vi "Experiment header-Get typedef cluster ref.vi"(7 "Header file sections":T22, 8 "error in (no error)":errorcluster, 11 "All header parameters / Header module interface cluster":refnum<vi>) -> (0 "error out":errorcluster, 1 "All header parameters in 2":refnum<vi>, 2 "Section Refs":T21[](array[typedef]), 3 "Controls[]":refnum<vi>[](array[refnum]))   [LabVIEW 2020]
uses:
  Typedefs/Header file sections.ctl
  Typedefs/Header file section refs.ctl
  Typedefs/Header parameters cluster-ALL.ctl
  Typedefs/Header subclusters/Header params -Login.ctl
  Typedefs/Header subclusters/Header params-Global Parameters.ctl
  Misc/Experiment Type.ctl
  Typedefs/Header subclusters/Header params-Imaging Modes.ctl
  Typedefs/Header subclusters/Header params-Time Series.ctl
  Typedefs/Header subclusters/Header params-Basic image meta data.ctl
  Typedefs/Frame Size.ctl
  Typedefs/Header subclusters/Header params-Motor Z-stack.ctl
  Typedefs/Header subclusters/Header params-AOL Z-stack.ctl
  Typedefs/Header subclusters/Header params-Functional Imaging.ctl
  Typedefs/Functional Mode.ctl
  Typedefs/AOL modes.ctl
  Typedefs/Plane Mode.ctl
  Typedefs/Header subclusters/Header params-Movement correction.ctl
  Typedefs/Reference source.ctl
  Typedefs/Header subclusters/Header params-Calibration Setup.ctl
  Typedefs/Header subclusters/Header params-statistics.ctl
  Misc/Biology Information.ctl
  Typedefs/Header subclusters/Header params-calibration data.ctl
panel:
  in  "All header parameters in":T1 {"VOLUME IMAGING"."Plane Mode" items=["XY Plane", "XZ Plane", "YZ Plane", "arbitraryplane"]; "VOLUME IMAGING"."Basic Image meta data"."Frame Size" items=["100X100"=100, "128X128"=128, "200X200"=200, "256X256"=256, "512X512"=512, "1024x1024"=1024, "2048x2048"=2048]; "AOL Z-STACK"."Hdr Basic Image meta data"."Frame Size" items=["100X100"=100, "128X128"=128, "200X200"=200, "256X256"=256, "512X512"=512, "1024x1024"=1024, "2048x2048"=2048]; "MOTOR Z-STACK"."Hdr Basic Image meta data"."Frame Size" items=["100X100"=100, "128X128"=128, "200X200"=200, "256X256"=256, "512X512"=512, "1024x1024"=1024, "2048x2048"=2048]; "FUNCTIONAL IMAGING"."Plane Mode" items=["XY Plane", "XZ Plane", "YZ Plane", "arbitraryplane"]; "FUNCTIONAL IMAGING"."Basic Image meta data"."Frame Size" items=["100X100"=100, "128X128"=128, "200X200"=200, "256X256"=256, "512X512"=512, "1024x1024"=1024, "2048x2048"=2048]; "TIME SERIES"."Basic Image meta data"."Frame Size" items=["100X100"=100, "128X128"=128, "200X200"=200, "256X256"=256, "512X512"=512, "1024x1024"=1024, "2048x2048"=2048]}
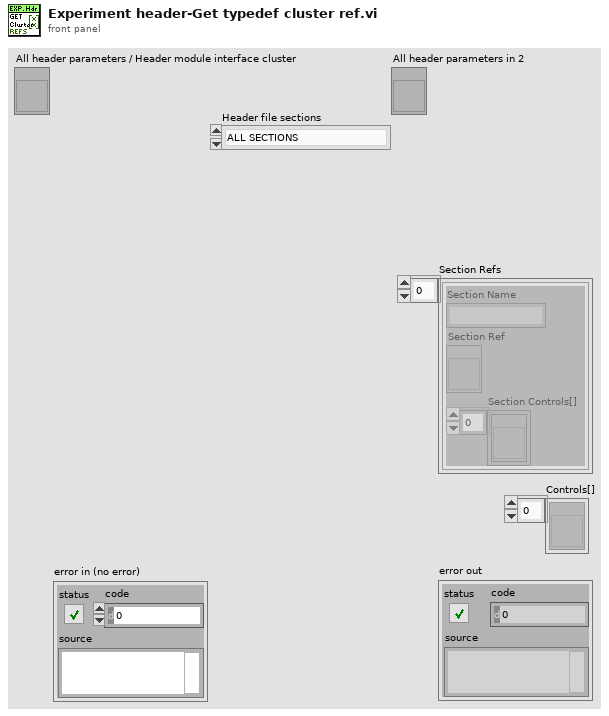
[diagram p1: front panel]
types:
  T1 = typedef "Header parameters cluster-ALL.ctl" = cluster{"LOGIN":T2, "GLOBAL PARAMETERS":T3, "IMAGING MODES":T5, "TIME SERIES":T6, "MOTOR Z-STACK ":T9, "AOL Z-STACK":T10, "FUNCTIONAL IMAGING":T11, "VOLUME IMAGING":T11, "MOVEMENT CORRECTION":T15, "CALIBRATION":T17, "STATISTICS":T18, "BIOLOGY INFORMATION":T19, "Calibration Data":T20}
  T2 = typedef "Header params -Login.ctl" = cluster{"User":string, "Profile":string, "Software Version":string, "Experiment Date Time":timestamp}
  T3 = typedef "Header params-Global Parameters.ctl" = cluster{"MicroscopeID":string, "Microscope Type":string, "Objective":string, "Field of View (um)":dbl, "Fill time (us)":dbl, "Experiment Type":T4, "Stimuli Trigger":bool, "Speed Logging":bool}
  T4 = typedef "Experiment Type.ctl" = enum16{"In vivo", "In vitro", "Testing", "Calibration", "Other"}
  T5 = typedef "Header params-Imaging Modes.ctl" = cluster{"Time Series":bool, "Motor Zstack":bool, "AOL Zstack":bool, "Functional Imaging":bool, "Volume Imaging":bool}
  T6 = typedef "Header params-Time Series.ctl" = cluster{"Basic Image meta data":T7, "AOL z":dbl}
  T7 = typedef "Header params-Basic image meta data.ctl" = cluster{"Wavelength (nm)":dbl, "# averaged frames":dbl, "laser power (%)":dbl, "Pockels":dbl, "pixel dwell time (us)":dbl, "pmt 1":dbl, "pmt 2":dbl, "back apperture":dbl, "zoom":dbl, "field of view":dbl, "Frame Size":T8, "AOL x centre":dbl, "AOL y centre":dbl, "Stage x position":dbl, "Stage y position":dbl, "Stage z position":dbl}
  T8 = typedef "Frame Size.ctl" = u16
  T9 = typedef "Header params-Motor Z-stack.ctl" = cluster{"Hdr Basic Image meta data":T7, "Z Start":dbl, "Z Stop":dbl, "No of Planes":i32, "Laser Power (%) at Z Start":dbl, "Laser Power (%) at Z Stop":dbl}
  T10 = typedef "Header params-AOL Z-stack.ctl" = cluster{"Hdr Basic Image meta data":T7, "Z Start":dbl, "Z Stop":dbl, "No of Planes":i32, "Laser Power (%) at Z Start":dbl, "Laser Power (%) at Z Stop":dbl}
  T11 = typedef "Header params-Functional Imaging.ctl" = cluster{"Functional Mode":T12, "Variable Length":bool, "Variable Resolution":bool, "Pockels Modulation":bool, "Stimuli Trigger":bool, "Cool down enabled":bool, "AOL Mode":T13, "Plane Mode":T14, "Miniscan Dwell time per pixel (us)":dbl, "poi dwell time":dbl, "Number of trials":dbl, "Number of cycles":dbl, "Number of pois":dbl, "Number of miniscans":dbl, "Number of pixels in miniscan":dbl, "Rectangle ROI length":dbl, "Rectangle ROI height":dbl, "Frame rate (fps)":dbl, "Acquisition Length":dbl, "video length (sec)":dbl, "Stimuli delay (sec)":dbl, "Cool down time (sec)":dbl, "Basic Image meta data":T7, "Z Start (um)":dbl, "Z Stop (um)":dbl}
  T12 = typedef "Functional Mode.ctl" = enum16{"Point", "Line", "Patch", "Plane", "Volume"}
  T13 = typedef "AOL modes.ctl" = enum16{"Raster", "Structural", "Pointing", "Mini Scan", "Alignment"}
  T14 = typedef "Plane Mode.ctl" = u16
  T15 = typedef "Header params-Movement correction.ctl" = cluster{"Movement Correction":bool, "Axial Reference":bool, "Reference Source":T16, "Full Frame Size":dbl, "Reference Field of View":dbl, "Reference Zoom":dbl, "Reference dwell time (us)":dbl, "Reference X Pixels":dbl, "Reference Y Pixels":dbl, "Number of Z lines":dbl, "Size of Z pixels":dbl, "Axial Pixels":dbl, "Ignore Z lines":dbl, "Reference Scan Cycles":dbl, "Reference Threshold XY":dbl, "Reference Threshold Z":dbl, "Reference Average XY":dbl, "Reference Average Z":dbl, "Proportional Scale":dbl, "Integral Scale":dbl, "Proportional Scale Z":dbl, "Integral Scale Z":dbl, "Diff Threshold":dbl, "Diff Threshold Z":dbl, "Sliding Average":bool, "Reference count reset enabled":bool, "Scan Interval (ms)":dbl, "Ref Plot Refresh Rate (ms)":dbl}
  T16 = typedef "Reference source.ctl" = enum16{"Green channel", "Red channel"}
  T17 = typedef "Header params-Calibration Setup.ctl" = cluster{"Pockels Calibration File":path, "Calibration_ini file":path, "Setup_ini file":path}
  T18 = typedef "Header params-statistics.ctl" = cluster{"Z-stack duration (sec)":dbl, "Number of acquired data-points":dbl, "Acquisition time (ms)":dbl, "Number of acquired frames":dbl, "Intertrial times":dbl[]}
  T19 = typedef "Biology Information.ctl" = cluster{"Animal Code or Name":string, "Animal DoB":string, "Animal Age":string, "Animal Sex":string, "Animal Weight":string, "Date of Injection":string, "Date of Implant":string, "Site of Injection":string, "Animal Ear Notch":string, "AAV constructs":string, "Genetic background":string, "Optical reporter":string, "Region of brain imaged":string, "Other \ncomments":string}
  T20 = typedef "Header params-calibration data.ctl" = cluster{"Objective Name":string, "Calibration Wavelength":dbl, "Sum X":dbl, "Sum Y":dbl, "Diff X":dbl, "Diff Y":dbl, "Distortion Correction":dbl, " Z norm to um Scaling":dbl, " X norm to um Scaling":dbl}
  T21 = typedef "Header file section refs.ctl" = cluster{"Section Name":string, "Section Ref":refnum<vi>, "Section Controls[]":refnum<vi>[]}
  T22 = typedef "Header file sections.ctl" = enum16{"ALL SECTIONS", "LOGIN", "GLOBAL PARAMETERS", "CALIBRATION DATA", "IMAGING MODES", "TIME SERIES", "MOTOR Z-STACK", "AOL Z-STACK", "FUNCTIONAL IMAGING", "VOLUME IMAGING", "ARBOREAL SCANNING", "MULTIBEAM PARAMETERS", "MOVEMENT CORRECTION", "CALIBRATION", "STATISTICS", "BIOLOGY INFORMATION", "PARAMETER SWEEP"}
  T23 = cluster{"Label.Text":string, refnum<vi>, "Controls OUT":refnum<vi>[]}
  T24 = cluster{"Label.Text":string, refnum<vi>, "Controls OUT":refnum<vi>[]}[]
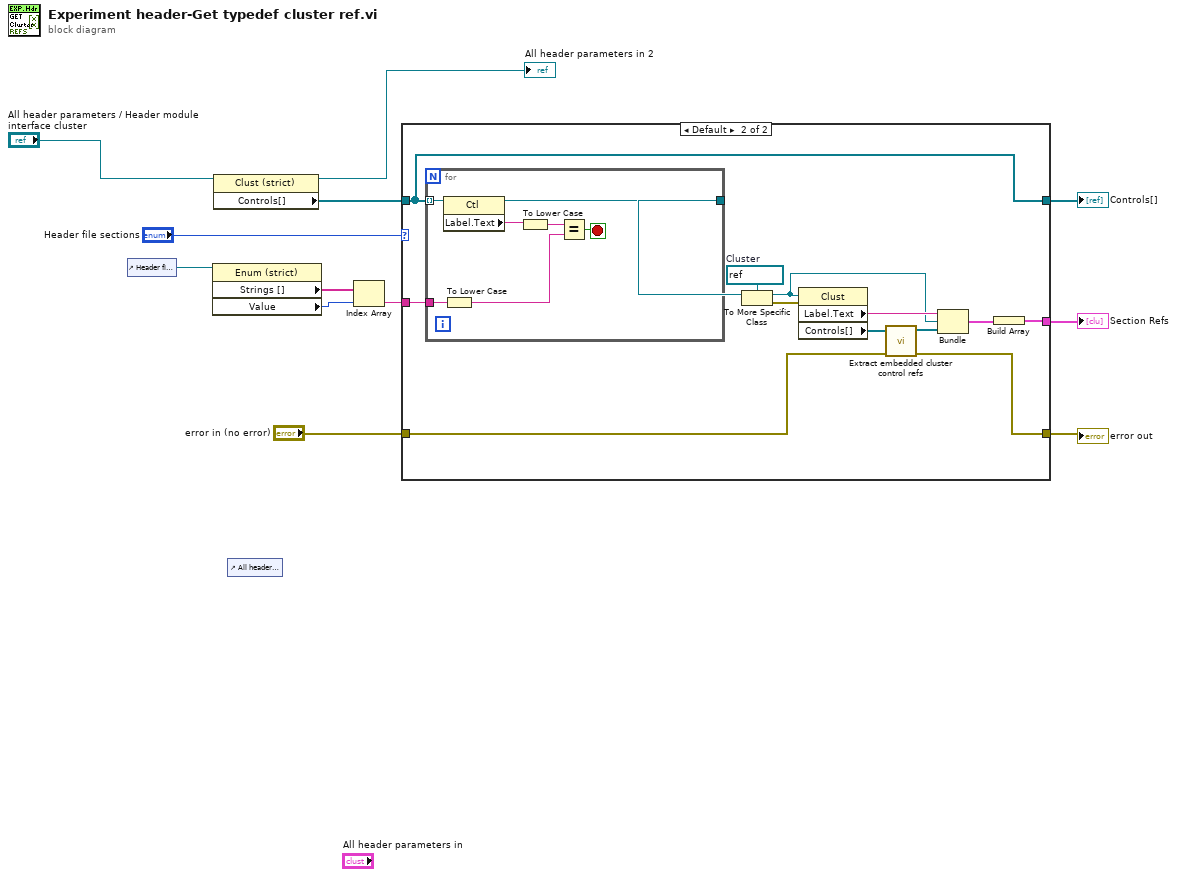
[diagram p0: block diagram]
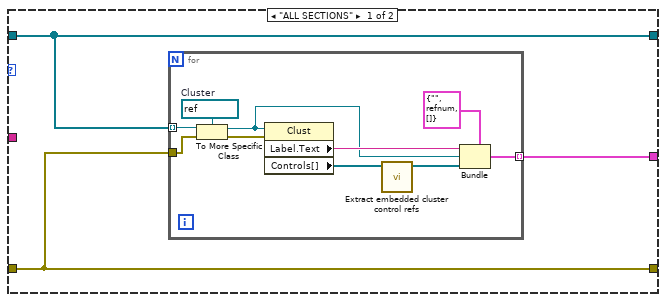
[diagram p2: hidden frame]
diagram:
  n1 = control-ref of="Header file sections"() -> (w9:refnum<vi>)
  n2 = property on="Property Node" class="Enum (strict)"(reference=w9) -> ("Strings []"=w8:string[], "Value"=w7:T22)  [unwired: 1 in, 2 out]
  n3 = property on="Property Node" class="Clust (strict)"(reference="All header parameters / Header module interface cluster") -> (reference out=→"All header parameters in 2":refnum<vi>, "Controls[]"=w11:refnum<vi>[])  [unwired: 1 in, 1 out]
  n4 = control-ref of="All header parameters in"() -> ()  [unwired: 1 out]
  n5 = Index Array(array=w8, index=w7) -> (element=w6:string)
  n6 = case shown="Default" "Header file sections" {
    tunnel: w11 -> [w15 w37]
    tunnel: [w15 w37] -> w10
    tunnel: w6 -> [_ w38]
    tunnel: "error in (no error)" -> [w14 w27]
    tunnel: [w14 w26] -> w4
    tunnel: [w13 w30] -> w3
    frame "ALL SECTIONS" {
      n7 = for {
        tunnel: w15 -> [w25] mode=indexing
        tunnel: w14 -> [w22]
        tunnel: [w19] -> w13 mode=indexing
        w24 = refnum<vi> refnum  # Cluster
        n8 = To More Specific Class(target class=w24, reference=w25, error in=w22) -> (specific class reference=w20:refnum<vi>, error out=w23:errorcluster)
        n9 = property on="Property Node" class="Clust"(reference=w20, error in=w23) -> ("Label.Text"=w21:string, "Controls[]"=w17:refnum<vi>[])  [unwired: 2 out]
        n10 = call "Extract embedded cluster control refs.vi"("Controls IN"=w17) -> ("Controls OUT"=w16:refnum<vi>[])  [unwired: 9 in, 1 out]
        n11 = Bundle(cluster=T21 {"Section Name"="", "Section Ref"=refnum, "Section Controls[]"=[]}, "Section Name"=w21, "Section Ref"=w20, "Section Controls[]"=w16) -> (w19:T21)
      }
    }
    frame Default {
      w36 = refnum<vi> refnum  # Cluster
      n12 = for {
        tunnel: w37 -> [w45] mode=indexing
        tunnel: w38 -> [w43]
        tunnel: [w39] -> w32
        stop <- w42 stop-if-true
        n13 = property on="Property Node" class="Ctl"(reference=w45) -> (reference out=w39:refnum<vi>, "Label.Text"=w44:string)  [unwired: 1 in, 1 out]
        n14 = To Lower Case(string=w43) -> (all lower case string=w41:string)
        n15 = To Lower Case(string=w44) -> (all lower case string=w40:string)
        n16 = Equal?(x=w40, y=w41) -> (x = y?=w42:bool)
      }
      n17 = To More Specific Class(target class=w36, reference=w32) -> (specific class reference=w33:refnum<vi>, error out=w35:errorcluster)  [unwired: 1 in]
      n18 = property on="Property Node" class="Clust"(reference=w33, error in=w35) -> ("Label.Text"=w34:string, "Controls[]"=w29:refnum<vi>[])  [unwired: 2 out]
      n19 = call "Extract embedded cluster control refs.vi"("error in (no error)"=w27, "Controls IN"=w29) -> ("error out"=w26:errorcluster, "Controls OUT"=w28:refnum<vi>[])  [unwired: 8 in]
      n20 = Bundle("Label.Text"=w34, w33, "Controls OUT"=w28) -> (w31:T23)  [unwired: 1 in]
      n21 = Build Array(w31) -> (w30:T24)
    }
  }
  "Controls[]" <- w10
  "error out" <- w4
  "Section Refs" <- w3
